vi "Determine Clicked Array Element Index - Is Array Element Gap Displayed.vi"(0 "Array Reference":refnum<vi>, 1 "Array Min Properties.Bounds.Width":u32, 3 "Array Min Properties.Position":T1, 5 "error in (no error)":errorcluster) -> (14 "dup Array Reference":refnum<vi>, 15 "Column Left Coordinates":i32[](array[numeric]), 16 "Row Top Coordinates":i32[](array[numeric]), 17 "Array has element gap?":bool, 18 "Un-gapped left coordinates":i32[](array[numeric]), 19 "error out":errorcluster)   [LabVIEW 2011]
doc: "Determine Clicked Array Element Index - Is Array Element Gap Displayed.vi\n\nDescription:\nThis VI calculates the gapped and un-gapped array element coordinates, determines if the array specified by the Array Reference input has an element gap displayed and outputs either the gapped or un-gapped coordinates accordingly.\n\nInputs:\nArray Reference - Reference to the array to operate on.\n\nArray Properties.Bounds.Width - The width of the array when the scrollbars, index display, label and caption are hidden.\n\nArray Min Properties.Position - The array position when the scrollbars, index display, label and caption are hidden.\n\nerror in - Standard error cluster.\n\nOutputs:\ndup Array Reference - Dup reference to the array to operate on.\n\nColumn left coordinates - The left coordinates of all columns displayed in the array.\n\nRow Top coordinates - The top coordinates of all rows displayed in the array.\n\nArray has element gap? - Indicates if the array has an element gap displayed or not.\n\nUn-gapped left coordinates - The calculated un-gapped coordinates.\n\nerror out - Standard error cluster.\n\nDeveloped By:\nMark.ridgley\nMark.Ridgley_LabVIEW.Developer@comcast.net"
uses:
  <vilib>/Utility/miscctls.llb/LVPositionTypeDef.ctl
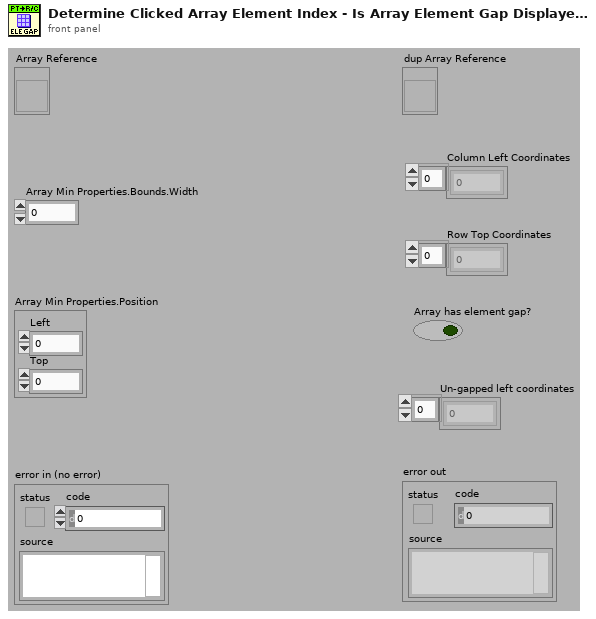
[diagram p1: front panel]
types:
  T1 = typedef "LVPositionTypeDef.ctl" = cluster{"Left":i32, "Top":i32}
  T2 = enum16{"Calculate Row Coordinates", "Calculate Col Coordinates"}
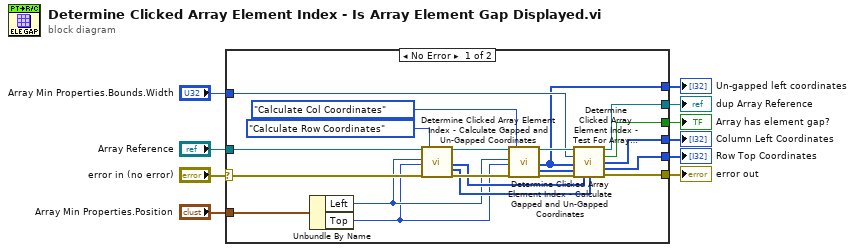
[diagram p0: block diagram]
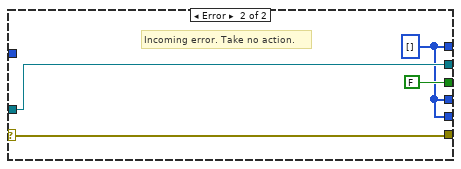
[diagram p2: hidden frame]
diagram:
  n1 = case shown="No Error" "error in (no error)" {
    selector: "error in (no error)" -> [w30 w34]
    tunnel: "Array Min Properties.Bounds.Width" -> [w26 _]
    tunnel: "Array Reference" -> [w25 w33]
    tunnel: [w22 w32] -> w8
    tunnel: "Array Min Properties.Position" -> [w18 _]
    tunnel: [w17 w32] -> w6
    tunnel: [w16 w32] -> w5
    tunnel: [w15 FALSE ("Array has element gap?")] -> w4
    tunnel: [w14 w34] -> w3
    tunnel: [w13 w33] -> w2
    frame No Error {
      n2 = Unbundle By Name(w18) -> ("Left"=w12:i32, "Top"=w11:i32)
      n3 = call "Determine Clicked Array Element Index - Calculate Gapped and Un-Gapped Coordinates.vi"("Array Reference"=w25, "Array Min Properties.Position.Left"=w12, "Array Min Properties.Position.Top"=w11, "error in (no error)"=w30, "Select Item"=T2."Calculate Row Coordinates") -> ("dup Array Reference"=w23:refnum<vi>, "Un-gapped coordinates"=w27:i32[], "Gapped coordinates"=w28:i32[], "error out"=w29:errorcluster)  [unwired: 11 in]
      n4 = call "Determine Clicked Array Element Index - Calculate Gapped and Un-Gapped Coordinates.vi"("Array Reference"=w23, "Array Min Properties.Position.Left"=w12, "Array Min Properties.Position.Top"=w11, "error in (no error)"=w29, "Select Item"=T2."Calculate Col Coordinates") -> ("dup Array Reference"=w31:refnum<vi>, "Un-gapped coordinates"=w22:i32[], "Gapped coordinates"=w20:i32[], "error out"=w24:errorcluster)  [unwired: 11 in]
      n5 = call "Determine Clicked Array Element Index - Test For Array Element Gap.vi"("Array Reference"=w31, "Array Property.Bounds.Width"=w26, "Un-gapped left coordinates"=w22, "Gapped left coordinates"=w20, "error in (no error)"=w24, "Un-gapped top coordinates"=w27, "Gapped top coordinates"=w28) -> ("dup Array Reference"=w13:refnum<vi>, "Array has element gap?"=w15:bool, "Column Left Coordinates"=w16:i32[], "Row Top Coordinates"=w17:i32[], "error out"=w14:errorcluster)  [unwired: 4 in]
    }
    frame Error {
      w32 = i32[] [] ("Un-gapped coordinates")
      # "Incoming error. Take no action."
    }
  }
  "Un-gapped left coordinates" <- w8
  "Row Top Coordinates" <- w6
  "Column Left Coordinates" <- w5
  "Array has element gap?" <- w4
  "dup Array Reference" <- w2
  "error out" <- w3
